vi "Display.vi"() -> ()   [LabVIEW 2020]
panel:
  out "High temperature":bool
  out "Trend":dbl
  out "TimeDisplay":string
  out "TempChart":dbl(graph)
  in  "Stop":bool
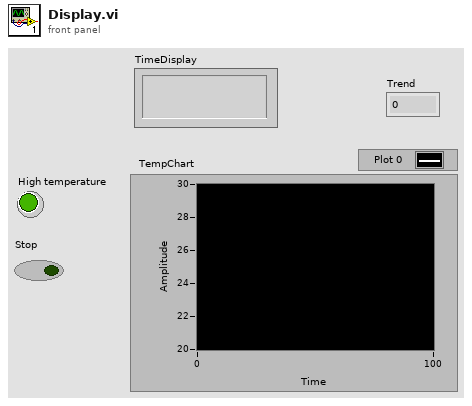
[diagram p1: front panel]
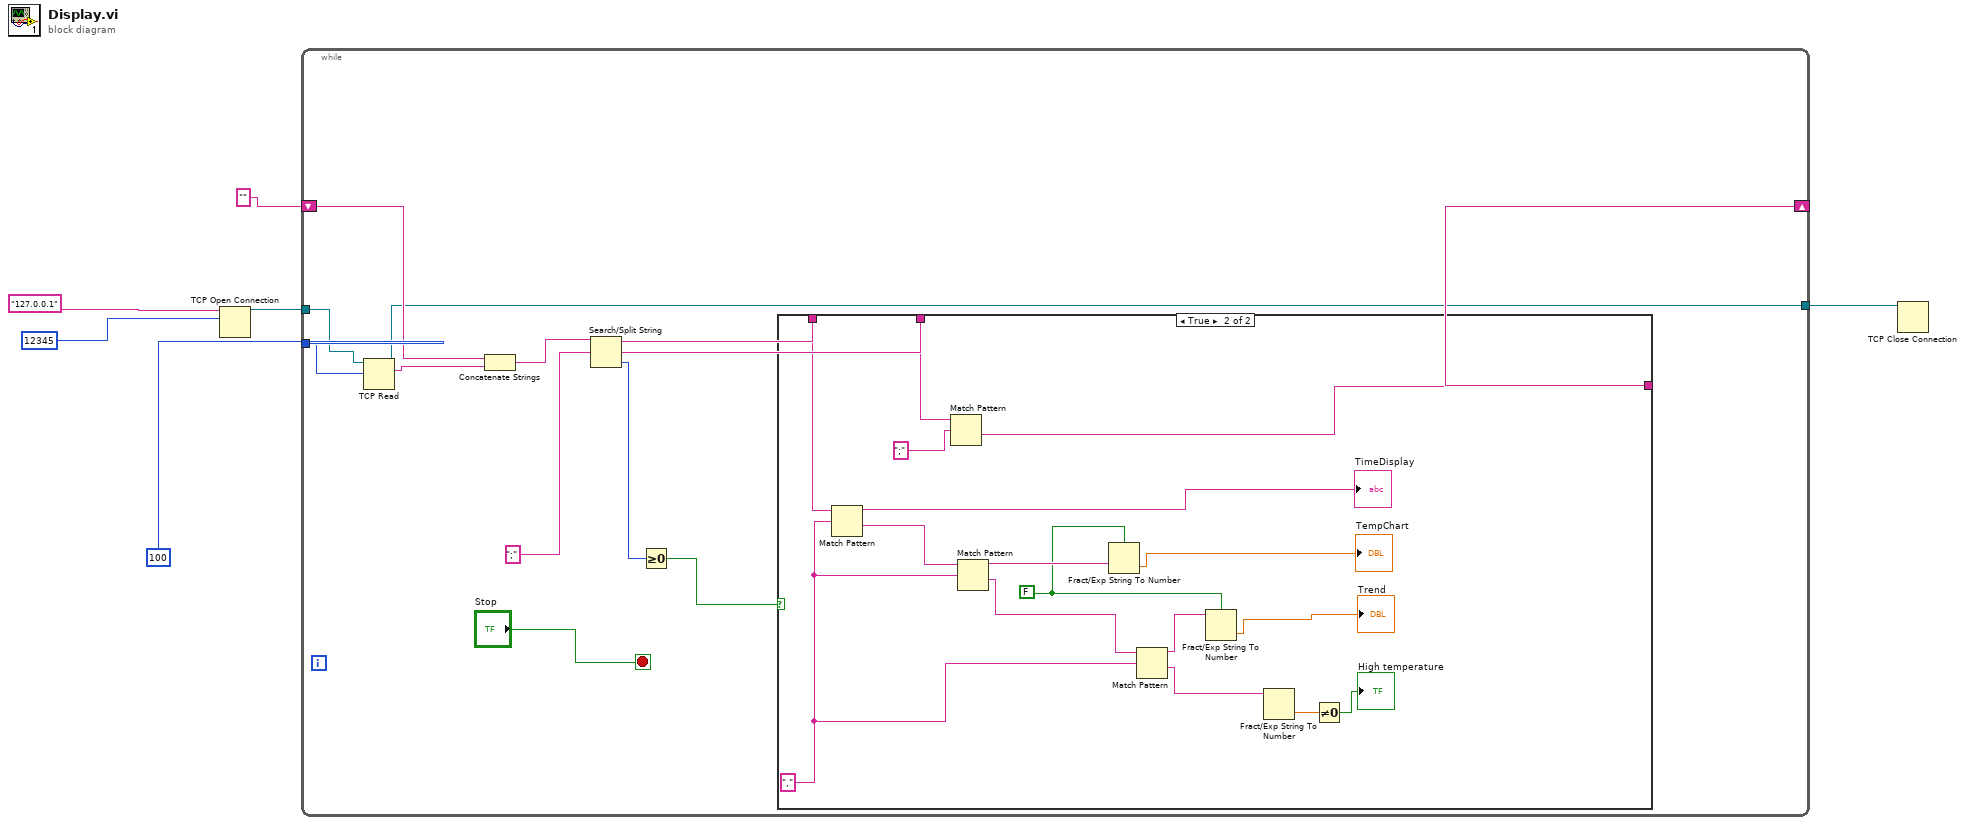
[diagram p0: block diagram]
diagram:
  n1 = TCP Open Connection(address="127.0.0.1", remote port or service name=12345) -> (connection ID=w5:refnum<k5>)  [unwired: 3 in, 1 out]
  n2 = while {
    tunnel: w5 -> [w9]
    tunnel: 100 -> [w10]
    tunnel: [w7] -> w3
    shift-right: [w13] -> _
    shift-left: "" -> [w18]
    stop <- "Stop" stop-if-true
    n3 = TCP Read(connection ID=w9, bytes to read=w10) -> (connection ID out=w7:refnum<k5>, data out=w8:string)  [unwired: 3 in, 1 out]
    n4 = Concatenate Strings(w18, w8) -> (w16:string)
    n5 = Search/Split String(string=w16, search string/char (-)=";") -> (substring before match=w12:string, match + rest of string=w11:string, offset of match=w15:i32)  [unwired: 1 in]
    n6 = Greater Or Equal To 0?(x=w15) -> (x >= 0?=w14:bool)
    n7 = case shown="True" w14 {
      tunnel: [w20 w32] -> w13
      tunnel: w12 -> [w20 w35]
      tunnel: w11 -> [_ w33]
      frame False {
      }
      frame True {
        w27 = FALSE
        w26 = ","
        n8 = Match Pattern(string=w35, regular expression=w26) -> (before substring=→"TimeDisplay":string, after substring=w31:string)  [unwired: 1 in, 2 out]
        n9 = Match Pattern(string=w33, regular expression=";") -> (after substring=w32:string)  [unwired: 1 in, 3 out]
        n10 = Match Pattern(string=w31, regular expression=w26) -> (before substring=w30:string, after substring=w25:string)  [unwired: 1 in, 2 out]
        n11 = Fract/Exp String To Number(use system decimal point (T)=w27, string=w30) -> (number=→"TempChart":dbl)  [unwired: 2 in, 1 out]
        n12 = Match Pattern(string=w25, regular expression=w26) -> (before substring=w24:string, after substring=w23:string)  [unwired: 1 in, 2 out]
        n13 = Fract/Exp String To Number(use system decimal point (T)=w27, string=w24) -> (number=→"Trend":dbl)  [unwired: 2 in, 1 out]
        n14 = Fract/Exp String To Number(string=w23) -> (number=w21:dbl)  [unwired: 3 in, 1 out]
        n15 = Not Equal To 0?(x=w21) -> (x != 0?=→"High temperature":bool)
      }
    }
  }
  n16 = TCP Close Connection(connection ID=w3) -> ()  [unwired: 2 in, 2 out]
